vi "SubVI Tester.vi"() -> ()   [LabVIEW 2012]
panel:
  out "Weather Data":T1={"Current Temp"=29.937499999999993, "Max Temp"=30.0, "Min Temp"=10.0, "Warning?"=FALSE, "Warning Text"="No Warning"}
  in  "Min Temp":dbl=10.0
  in  "Max Temp":dbl=30.0
  in  "Stop":bool
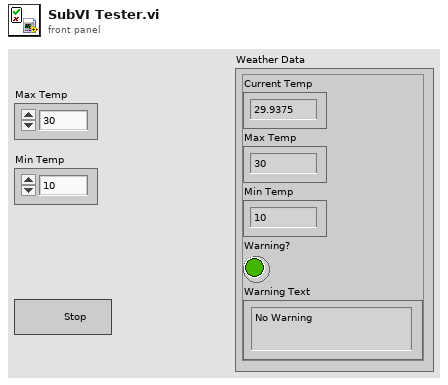
[diagram p1: front panel]
types:
  T1 = cluster{"Current Temp":dbl, "Max Temp":dbl, "Min Temp":dbl, "Warning?":bool, "Warning Text":string}
  T2 = cluster{"Current Temperature":dbl, "Max Temperature":dbl, "Min Temperature":dbl, "Warning?":bool, "Warning Text":string}
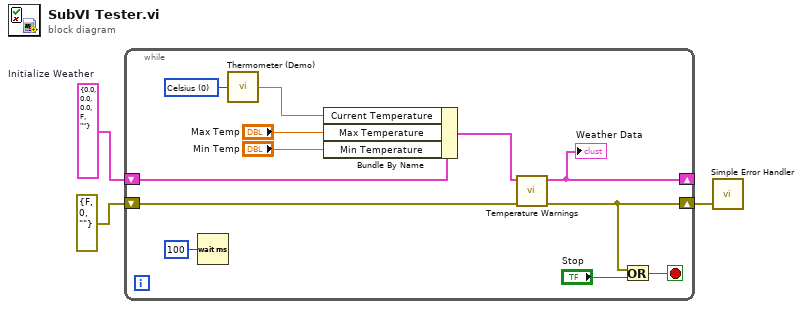
[diagram p0: block diagram]
diagram:
  w3 = T2 {"Current Temperature"=0.0, "Max Temperature"=0.0, "Min Temperature"=0.0, "Warning?"=FALSE, "Warning Text"=""}  # Initialize Weather
  n1 = while {
    shift-right: [w10] -> _
    shift-left: w3 -> [w4]
    shift-right: [w11] -> w2
    shift-left: errorcluster {"status"=FALSE, "code"=0, "source"=""} ("error out") -> [w12]
    stop <- w13 stop-if-true
    w9 = u16 0 items=["Celsius", "Fahrenheit"] ("Units (0: Celsius)")
    n2 = Wait (ms)(milliseconds to wait=u32 100) -> ()  [unwired: 1 out]
    n3 = call "Thermometer (Demo).vi"("Units (0: Celsius)"=w9) -> ("Temperature Value"=w6:dbl)
    n4 = Bundle By Name(cluster=w4, "Current Temperature"=w6, "Max Temperature"="Max Temp", "Min Temperature"="Min Temp") -> (w5:T2)
    n5 = call "Temperature Warnings.vi"("Error In"=w12, "Weather Data In"=w5) -> ("Error Out"=w11:errorcluster, "Weather Data Out"=w10:T2)  [unwired: 8 in]
    "Weather Data" <- w10
    n6 = Or(x=w11, y="Stop") -> (x .or. y?=w13:bool)
  }
  n7 = call <vilib>:"Simple Error Handler.vi"("error in (no error)"=w2) -> ()  [unwired: 4 in, 5 out]
